vi "Measurement Logic Debug.vi"(8 "error in":errorcluster, 9 "measurement configuration":T4={"SERIAL CHANNEL"="SI1", "PATH TO CONFIGURATION SCRIPT"="\"C:\\dev\\scripts\\Image Receiver Scripts\\9296A_RAW8.cpp\"", "REF. CLOCK  (Hz)"=25000000.0, "POC SOURCE"=0, "CSI-2 DATA SOURCE"=0, "SI ACTIVE LANE CNT"=4, "PAYLOAD DATA TYPE"=enum."RAW 8", "INTERPRETATION"=1, "VIRTUAL CHANNEL"=0, "PATTERN"=0, "ALGORITHM"=0, "RIO HANDLER"="PXI1Slot2", "AUTO. VISION DEVICE"=0, "SERIAL (SI) CHANNEL"=1, "BITFILE"="PXIe_1487_4_In_4_Out_Acq_Tap.lvbitx", "SI CHANNELS"="SI0, S01"} {"SERIAL (SI) CHANNEL" items=["SI0", "SI1"]; "AUTO. VISION DEVICE" items=["PXI1Slot2", "PXI1Slot5"]; "ALGORITHM" items=["BILINEAR", "VNG"]; "PATTERN" items=["GB", "GR", "BG", "RG"]; "INTERPRETATION" items=["Grayscale", "Bayer", "RGB", "YUV422", "YUV420", "Legacy YUV420"]; "SI ACTIVE LANE CNT" items=["1 LANE"=1, "2 LANE"=2, "4 LANE"=4]; "CSI-2 DATA SOURCE" items=["CORRECTED", "RAW"]; "POC SOURCE" items=["NONE", "INTERNAL", "AUXILIARY"]}, 10 "measure call context in":refnum<class "Measure Call Context.lvclass">, 11 "user event out":refnum<user-event>) -> (0 "Error Out":errorcluster, 2 "measure call context out":refnum<class "Measure Call Context.lvclass">, 3 "measurement results":T1 {"BYTES ACQUIRED" format="%#.6p"})   [LabVIEW 2025]
doc: "Contains the core logic for executing the measurement."
uses:
  <vilib>/Plug-In SDKs/Measurements/Measure Call Context/Measure Call Context.lvclass
  <vilib>/rvi/interface/nirviCloseFPGA/nirviCloseFPGA.xnode
  Measurement Results.ctl
  Automotive Vision.lvclass
  deps/NI148X/Getting Started/Host/Acq/GettingStarted_Acq_148X_Host.lvlib
  deps/NI148X/Getting Started/Host/Common/GettingStarted_Common_148X_Host.lvlib
  <instrlib>/FlexRIO/API/Host/v1/NI FlexRIO API v1.lvlib
  <vilib>/vision/Image Controls.llb/IMAQ Image.ctl
  <instrlib>/FlexRIO/CSI-2/v2/Common/Types/LLP Data Type.ctl
  <instrlib>/FlexRIO/CSI-2/v2/Common/NI CSI-2 API Common v2.lvlib
  <instrlib>/FlexRIO/API/Host/v1/NI FlexRIO/API/Wait for PoC Safe to Disconnect Channels Array.vi
  <vilib>/FPGAPlugInAG/Dynamic/niLvFpga_Close_Dynamic.vi
  Measurement Configuration.ctl
panel:
  in  "Acquired Serial Input Channel Data":T2(tab)
  out "Source Rate (fps)(1st Display)":dbl
  out "Update Rate (fps)(1st Display)":dbl
  out "1st channel display":T3(plugin-control)
  out "Bytes Acquired (1st Channel)":i64 format="%#.6p"
  out "Packets Logged (1st Channel)":i64
  out "Source Rate (fps)(2nd Display)":dbl
  out "Update Rate (fps)(2nd Display)":dbl
  out "2nd channel display":T3(plugin-control)
  out "Packets Logged (2nd Channel)":i64
  out "Bytes Acquired (2nd Channel)":i64 format="%#.6p"
  out "Acquisition In Progress":bool
  out "Acquisition Duration (s)":dbl format="%.1f"
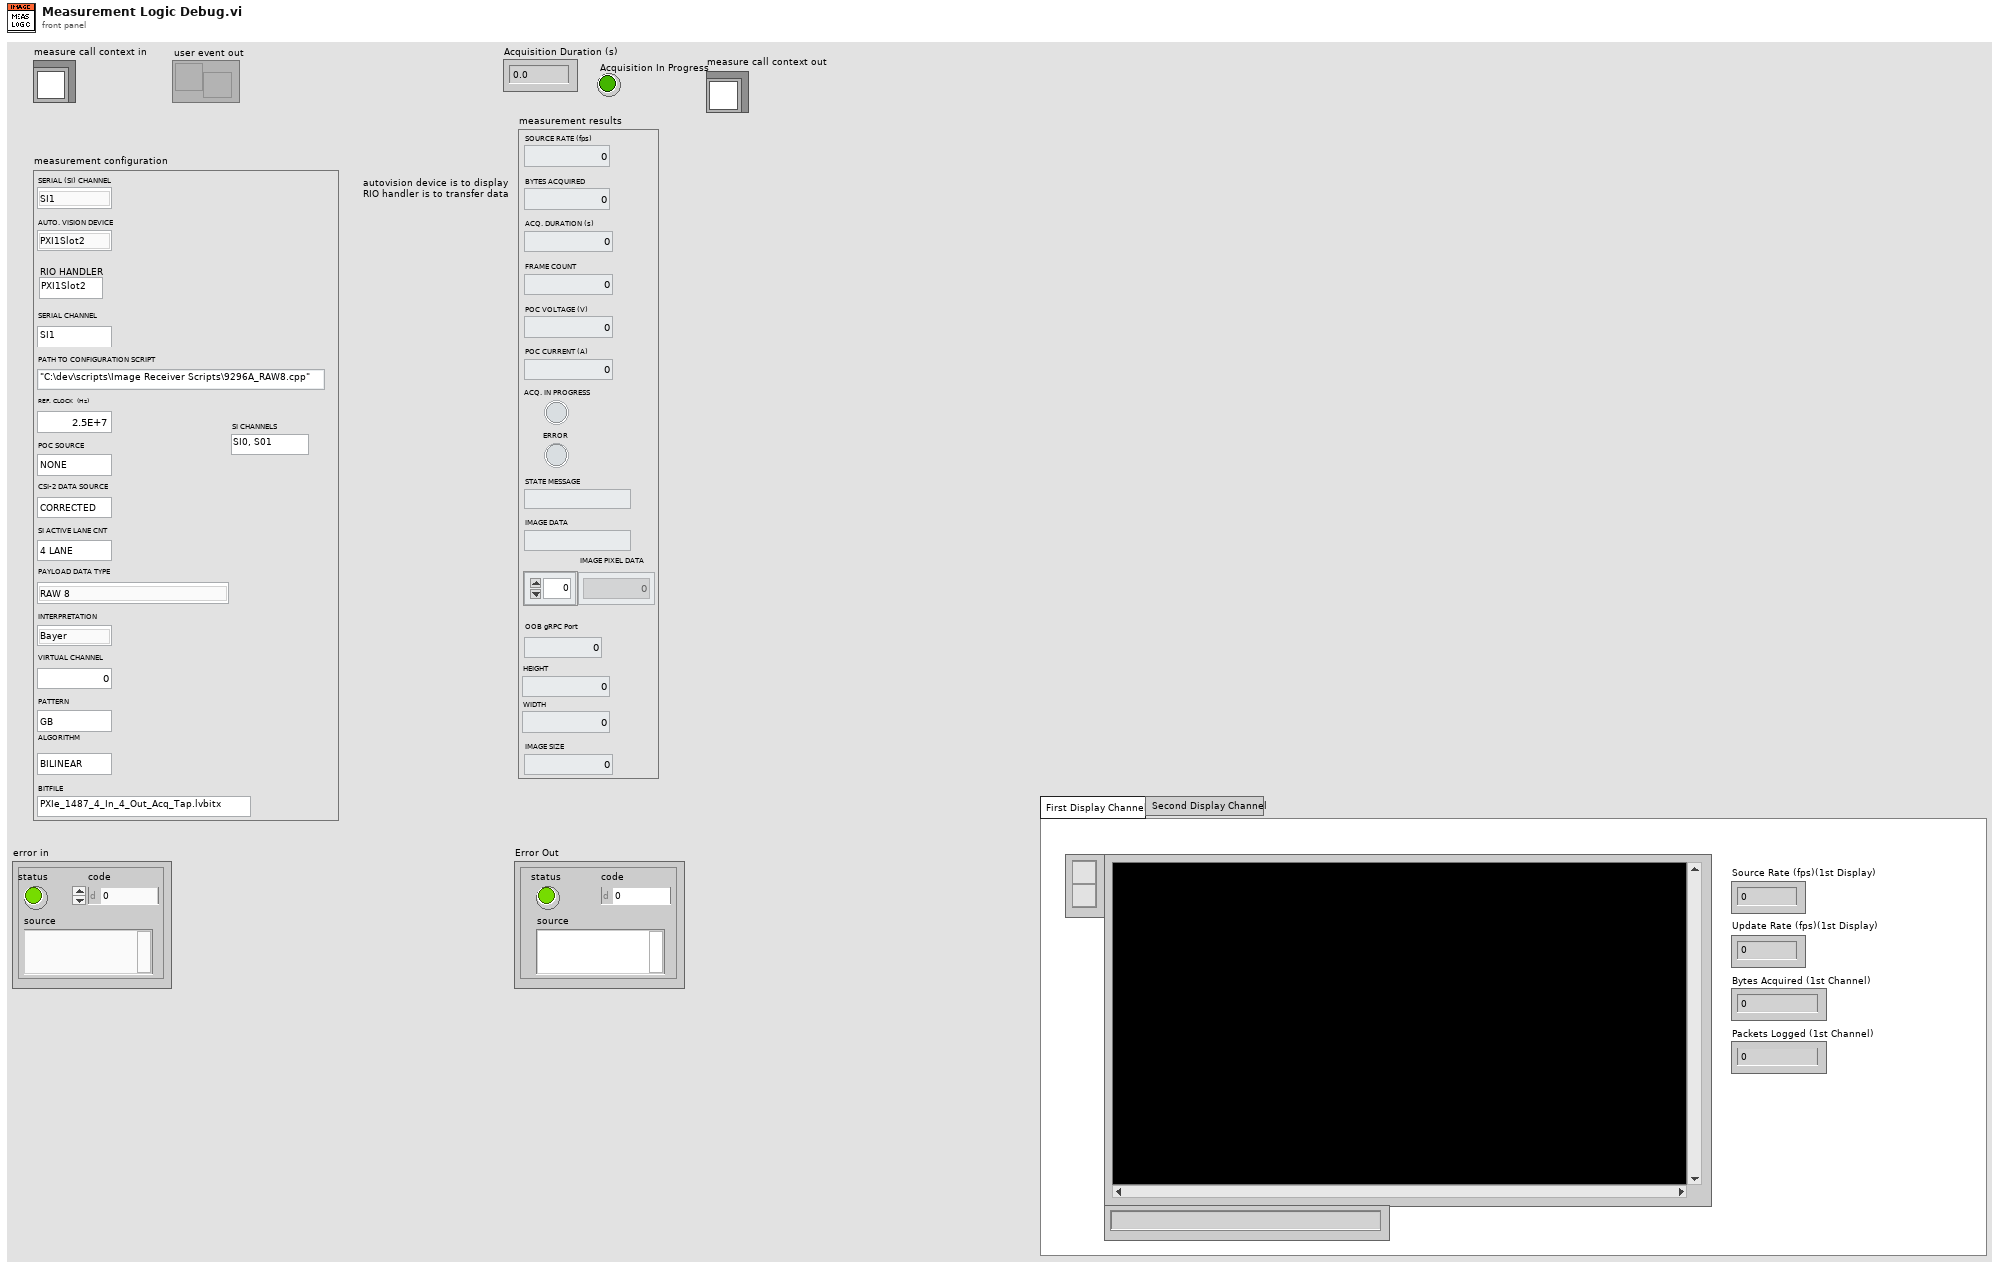
[diagram p1: front panel]
types:
  T1 = typedef "Automotive Vision.lvclass/Measurement Results.ctl" = cluster{"ACQ. IN PROGRESS":bool, "IMAGE PIXEL DATA":u32[], "ACQ. DURATION (s)":dbl, "SOURCE RATE (fps)":dbl, "BYTES ACQUIRED":u64, "FRAME COUNT":u64, "POC VOLTAGE (V)":dbl, "POC CURRENT (A)":dbl, "ERROR":bool, "STATE MESSAGE":string, "IMAGE DATA":string, "OOB gRPC Port":i32, "HEIGHT":u64, "WIDTH":u64, "IMAGE SIZE":u64}
  T2 = enum32{"First Display Channel", "Second Display Channel"}
  T3 = typedef "IMAQ Image.ctl" = refnum<image>
  T4 = typedef "Automotive Vision.lvclass/Measurement Configuration.ctl" = cluster{"SERIAL CHANNEL":string, "PATH TO CONFIGURATION SCRIPT":string, "REF. CLOCK  (Hz)":dbl, "POC SOURCE":u32, "CSI-2 DATA SOURCE":u32, "SI ACTIVE LANE CNT":u32, "PAYLOAD DATA TYPE":enum32{"Frame Start", "Frame End", "Line Start", "Line End", "End of Transmission", "Reserved 0", "Reserved 1", "Reserved 2", "Generic Short Packet 1", "Generic Short Packet 2", "Generic Short Packet 3", "Generic Short Packet 4", "Generic Short Packet 5", "Generic Short Packet 6", "Generic Short Packet 7", "Generic Short Packet 8", "Null", "Blanking Data", "Embedded 8-bit non Image Data", "Generic Long Packet 1", "Generic Long Packet 2", "Generic Long Packet 3", "Generic Long Packet 4", "Reserved 3", "YUV420 8-bit", "YUV420 10-bit", "Legacy YUV420 8-bit", "Reserved 4", "YUV420 8-bit Chroma Shifted", "YUV420 10-bit Chroma Shifted", "YUV422 8-bit", "YUV422 10-bit", "RGB444", "RGB555", "RGB565", "RGB666", "RGB888", "Reserved 5", "Reserved 6", "RAW 24", "RAW 6", "RAW 7", "RAW 8", "RAW 10", "RAW 12", "RAW 14", "RAW 16", "RAW 20", "User Defined 8-bit Data 1", "User Defined 8-bit Data 2", "User Defined 8-bit Data 3", "User Defined 8-bit Data 4", "User Defined 8-bit Data 5", "User Defined 8-bit Data 6", "User Defined 8-bit Data 7", "User Defined 8-bit Data 8", "USL Command", "Reserved 7", "Reserved 8", "Reserved 9", "Reserved 10", "Reserved 11", "Reserved 12", "LRTE EPD Spacer"}, "INTERPRETATION":u32, "VIRTUAL CHANNEL":u32, "PATTERN":u32, "ALGORITHM":u32, "RIO HANDLER":string, "AUTO. VISION DEVICE":u32, "SERIAL (SI) CHANNEL":u32, "BITFILE":string, "SI CHANNELS":string}
  T5 = typedef "NI CSI-2 API Common v2.lvlib/LLP Data Type.ctl" = enum8{"Frame Start", "Frame End", "Line Start", "Line End", "End of Transmission", "Reserved 0", "Reserved 1", "Reserved 2", "Generic Short Packet 1", "Generic Short Packet 2", "Generic Short Packet 3", "Generic Short Packet 4", "Generic Short Packet 5", "Generic Short Packet 6", "Generic Short Packet 7", "Generic Short Packet 8", "Null", "Blanking Data", "Embedded 8-bit non Image Data", "Generic Long Packet 1", "Generic Long Packet 2", "Generic Long Packet 3", "Generic Long Packet 4", "Reserved 3", "YUV420 8-bit", "YUV420 10-bit", "Legacy YUV420 8-bit", "Reserved 4", "YUV420 8-bit Chroma Shifted", "YUV420 10-bit Chroma Shifted", "YUV422 8-bit", "YUV422 10-bit", "RGB444", "RGB555", "RGB565", "RGB666", "RGB888", "Reserved 5", "Reserved 6", "RAW 24", "RAW 6", "RAW 7", "RAW 8", "RAW 10", "RAW 12", "RAW 14", "RAW 16", "RAW 20", "User Defined 8-bit Data 1", "User Defined 8-bit Data 2", "User Defined 8-bit Data 3", "User Defined 8-bit Data 4", "User Defined 8-bit Data 5", "User Defined 8-bit Data 6", "User Defined 8-bit Data 7", "User Defined 8-bit Data 8", "USL Command", "Reserved 7", "Reserved 8", "Reserved 9", "Reserved 10", "Reserved 11", "Reserved 12", "LRTE EPD Spacer"}
  T6 = typedef "GettingStarted_Common_148X_Host.lvlib/Serial Channel Configuration.ctl" = cluster{"Serial Channel":string, "FPGA Display Parameters":T7, "RAW Display Parameters":cluster{"Interpretation":T8, "Bayer Parameters":cluster{"Pattern":i32, "Algorithm":i32, "Red Gain":dbl, "Green Gain":dbl, "Blue Gain":dbl}}}
  T7 = typedef "NI CSI-2 API FPGA v2.lvlib/Display Parameters.ctl" = cluster{"virtual channel":fxp<+,4,4>, "payload data type":T5, "frame skip count":u16, "line skip count":u8, "pixel skip count":fxp<+,5,5>}
  T8 = typedef "GettingStarted_Common_148X_Host.lvlib/RAW Interpretation for Display.ctl" = enum16{"Grayscale", "Bayer", "RGB", "YUV422", "YUV420", "Legacy YUV420"}
  T9 = typedef "GettingStarted_Common_148X_Host.lvlib/Serial Channel Display Parameters.ctl" = cluster{"images":cluster{"grayscale":T3, "color":T3}, "RAW parameters":cluster{"interpretation":T8, "bayer parameters":cluster{"pattern":i32, "algorithm":i32, "red gain":dbl, "green gain":dbl, "blue gain":dbl}}}
  T10 = cluster{"Acquisition In Progress":refnum<vi>, "Acquisition Duration (s)":refnum<vi>, "Bytes Acquired (1st Channel)":refnum<vi>}
  T11 = typedef "Event Messenger-bool.lvlib/))Channel.ctl" = refnum<queue>
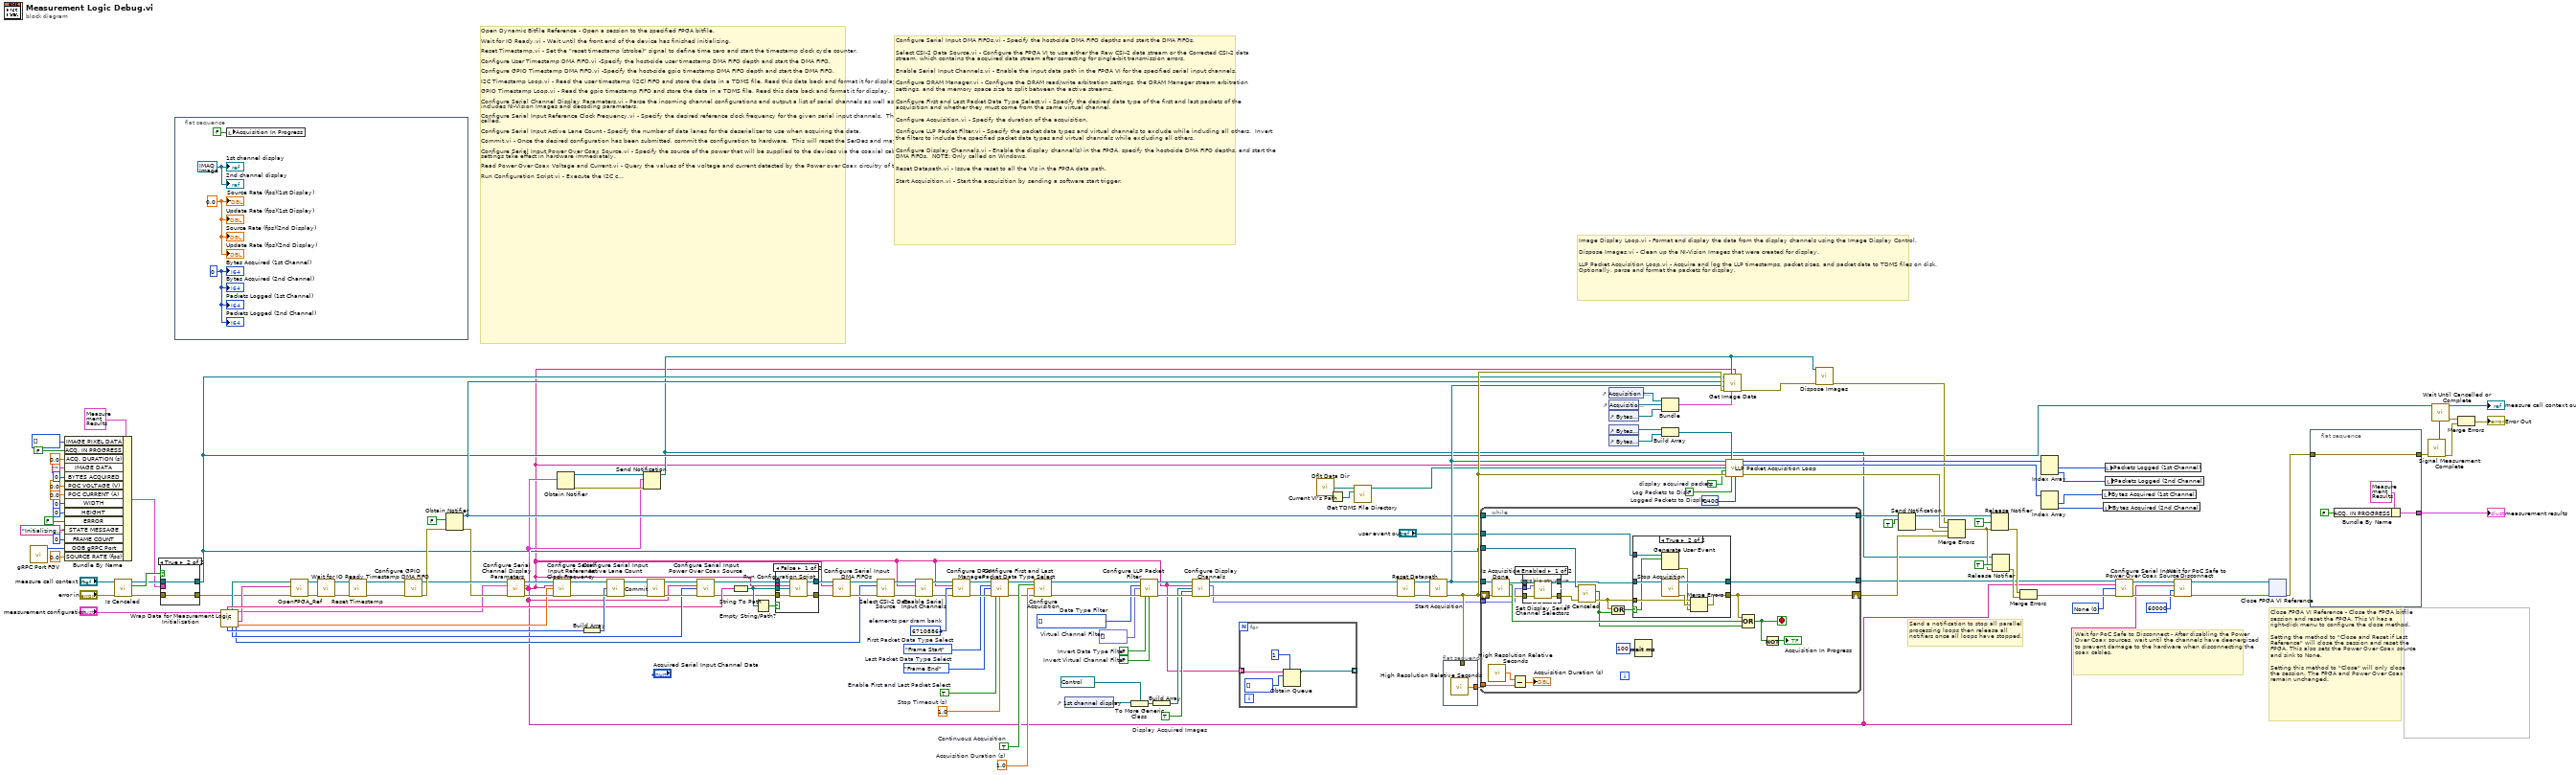
[diagram p0: block diagram]
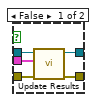
[diagram p2: hidden frame]
diagram:
  w78 = i64 1400  # Logged Packets to Display
  w102 = FALSE  # Log Packets to Disk
  w130 = FALSE  # Invert Virtual Channel Filter
  w131 = FALSE  # Invert Data Type Filter
  w132 = fxp<+,4,4>[] []  # Virtual Channel Filter
  w98 = TRUE  # Display Acquired Images
  w134 = T5[] [] items=["Frame Start", "Frame End", "Line Start", "Line End", "End of Transmission", "Reserved 0", "Reserved 1", "Reserved 2", "Generic Short Packet 1", "Generic Short Packet 2", "Generic Short Packet 3", "Generic Short Packet 4", "Generic Short Packet 5", "Generic Short Packet 6", "Generic Short Packet 7", "Generic Short Packet 8", "Null", "Blanking Data", "Embedded 8-bit non Image Data", "Generic Long Packet 1", "Generic Long Packet 2", "Generic Long Packet 3", "Generic Long Packet 4", "Reserved 3", "YUV420 8-bit", "YUV420 10-bit", "Legacy YUV420 8-bit", "Reserved 4", "YUV420 8-bit Chroma Shifted", "YUV420 10-bit Chroma Shifted", "YUV422 8-bit", "YUV422 10-bit", "RGB444", "RGB555", "RGB565", "RGB666", "RGB888", "Reserved 5", "Reserved 6", "RAW 24", "RAW 6", "RAW 7", "RAW 8", "RAW 10", "RAW 12", "RAW 14", "RAW 16", "RAW 20", "User Defined 8-bit Data 1", "User Defined 8-bit Data 2", "User Defined 8-bit Data 3", "User Defined 8-bit Data 4", "User Defined 8-bit Data 5", "User Defined 8-bit Data 6", "User Defined 8-bit Data 7", "User Defined 8-bit Data 8", "USL Command", "Reserved 7", "Reserved 8", "Reserved 9", "Reserved 10", "Reserved 11", "Reserved 12", "LRTE EPD Spacer"]  # Data Type Filter
  w137 = 1.0  # Acquisition Duration (s)
  w140 = TRUE  # Continuous Acquisition
  w120 = 1.0  # Stop Timeout (s)
  w121 = TRUE  # Enable First and Last Packet Select
  w118 = LLP_Data_Type."Frame End"  # Last Packet Data Type Select
  w119 = LLP_Data_Type."Frame Start"  # First Packet Data Type Select
  w59 = 0 items=["None", "Internal", "Auxiliary"] ("power over coax source")
  w79 = TRUE  # display acquired packets
  w146 = u32 67108864  # elements per dram bank
  # "Wait for PoC Safe to Disconnect - After disabling the Power Over Coax sources, wait until the channels have deenergized to prevent damage to the hardware when disconnecting the coax cables."
  # "Send a notification to stop all parallel processing loops then release all notifiers once all loops have stopped."
  # "Image Display Loop.vi - Format and display the data from the display channels using the Image Display Control.   \n\nDispose Images.vi - Clean up the NI-Vision Images that were created for display.\n\nLLP Packet Acquisition Loop.vi - Acquire and log the LLP timestamps, packet sizes, and packet data to TDMS files on disk.  Optionally, parse and format the packets for display."
  # "Configure Serial Input DMA FIFOs.vi - Specify the host-side DMA FIFO depths and start the DMA FIFOs.\n\nSelect CSI-2 Data Source.vi - Configure the FPGA VI to use either the Raw CSI-2 data stream or the Corrected CSI-2 data stream, which contains the acquired data stream after correcting for single-bit transmission errors.\n\nEnable Serial Input Channels.vi - Enable the input data path in the FPGA VI for the specified serial input channels.\n\nConfigure DRAM Manager.vi - Configure the DRAM read/write arbitration settings, the DRAM Manager stream arbitration settings, and the memory space size to split between the active streams.\n\nConfigure First and Last Packet Data Type Select.vi - Specify the desired data type of the first and last packets of the acquisition and whether they must come from the same virtual channel.\n\nConfigure Acquisition.vi - Specify the duration of the acquisition.\n\nConfigure LLP Packet Filter.vi - Specify the packet data types and virtual channels to exclude while including all others.  Invert the filters to include the specified packet data types and virtual channels while excluding all others.\n\nConfigure Display Channels.vi - Enable the display channel(s) in the FPGA, specify the host-side DMA FIFO depths, and start the DMA FIFOs.  NOTE: Only called on Windows. \n\nReset Datapath.vi - Issue the reset to all the VIs in the FPGA data path.\n\nStart Acquisition.vi - Start the acquisition by sending a software start trigger."
  # "Close FPGA VI Reference - Close the FPGA bitfile session and reset the FPGA. This VI has a right-click menu to configure the close method. \n\nSetting the method to \"Close and Reset if Last Reference\" will close the session and reset the FPGA. This also sets the Power Over Coax source and sink to None.\n\nSetting this method to \"Close\" will only close the session. The FPGA and Power Over Coax remain unchanged."
  # "Open Dynamic Bitfile Reference - Open a session to the specified FPGA bitfile.\n\nWait for IO Ready.vi - Wait until the front end of the device has finished initializing.\n\nReset Timestamp.vi - Set the \"reset timestamp (strobe)\" signal to define time zero and start the timestamp clock cycle counter.\n\nConfigure User Timestamp DMA FIFO.vi -Specify the host-side user timestamp DMA FIFO depth and start the DMA FIFO.\n\nConfigure GPIO Timestamp DMA FIFO.vi -Specify the host-side gpio timestamp DMA FIFO depth and start the DMA FIFO.\n\nI2C Timestamp Loop.vi - Read the user timestamp (I2C) FIFO and store the data in a TDMS file. Read this data back and format it for display.\n\nGPIO Timestamp Loop.vi - Read the gpio timestamp FIFO and store the data in a TDMS file. Read this data back and format it for display.\n\nConfigure Serial Channel Display Parameters.vi - Parse the incoming channel configurations and output a list of serial channels as well as a list of serial channel display parameters, which includes NI-Vision Images and decoding parameters.\n\nConfigure Serial Input Reference Clock Frequency.vi - Specify the desired reference clock frequency for the given serial input channels.  These settings do not take effect until Commit.vi is called.\n\nConfigure Serial Input Active Lane Count - Specify the number of data lanes for the deserializer to use when acquiring the data. \n\nCommit.vi - Once the desired configuration has been submitted, commit the configuration to hardware.  This will reset the SerDes and may cause GPIO lines to toggle. \n\nConfigure Serial Input Power Over Coax Source.vi - Specify the source of the power that will be supplied to the devices via the coaxial cables attached to the given serial input channels.  These settings take effect in hardware immediately.\n\nRead Power Over Coax Voltage and Current.vi - Query the values of the voltage and current detected by the Power over Coax circuitry of the given serial channels.\n\nRun Configuration Script.vi - Execute the I2C commands in the specified script file for the given serial channels.  The script is used to configure the serializer, deserializer, or other I2C slave device, such as the image sensor."
  n1 = call "gRPC Port FGV.vi"() -> ("Listening Port out"=w31:i32)  [unwired: 11 in]
  n2 = Bundle By Name(cluster=T1 {"ACQ. IN PROGRESS"=FALSE, "IMAGE PIXEL DATA"=[], "ACQ. DURATION (s)"=0.0, "SOURCE RATE (fps)"=0.0, "BYTES ACQUIRED"=0, "FRAME COUNT"=0, "POC VOLTAGE (V)"=0.0, "POC CURRENT (A)"=0.0, "ERROR"=FALSE, "STATE MESSAGE"="", "IMAGE DATA"="", "OOB gRPC Port"=0, "HEIGHT"=0, "WIDTH"=0, "IMAGE SIZE"=0} ("Measurement Results"), "IMAGE PIXEL DATA"=u32[] [], "ACQ. IN PROGRESS"=FALSE, "ACQ. DURATION (s)"=0.0, "IMAGE DATA"="", "BYTES ACQUIRED"=u64 0, "POC VOLTAGE (V)"=0.0, "POC CURRENT (A)"=0.0, "WIDTH"=u64 0, "HEIGHT"=u64 0, "ERROR"=FALSE, "STATE MESSAGE"="Initializing...", "FRAME COUNT"=u64 0, "OOB gRPC Port"=w31, "SOURCE RATE (fps)"=0.0) -> (w27:T1)
  n3 = call <vilib>:"Is Canceled.vi"("error in"="error in", "measure call context in"="measure call context in") -> ("error out"=w30:errorcluster, "is canceled?"=w29:bool, "measure call context out"=w28:refnum<class "Measure Call Context.lvclass">)  [unwired: 7 in]
  n4 = case shown="True" w29 {
    tunnel: w27 -> [w155 _]
    tunnel: [w154 w157] -> w24
    tunnel: w28 -> [w153 w156]
    tunnel: w30 -> [w152 w157]
    tunnel: [w151 w156] -> w9
    frame False {
      n5 = call <vilib>:"Update Results.vi"("error in"=w152, "measurement results"=w155, "measure call context in"=w153) -> ("error out"=w154:errorcluster, "measure call context out"=w151:refnum<class "Measure Call Context.lvclass">)  [unwired: 7 in]
    }
    frame True {
    }
  }
  n6 = flat-sequence {
    frame #0 {
      w159 = i64 0 ("Number of Packets Acquired (1st Channel)")
      w160 = 0.0 ("display fps (2nd display)")
      w161 = T3 refnum ("first channel display")
      n7 = local write "Acquisition In Progress"(FALSE ("Acquisition In Progress")) -> ()
      "1st channel display" <- w161
      "2nd channel display" <- w161
      "Update Rate (fps)(1st Display)" <- w160
      "Update Rate (fps)(2nd Display)" <- w160
      "Packets Logged (1st Channel)" <- w159
      "Packets Logged (2nd Channel)" <- w159
      "Source Rate (fps)(1st Display)" <- w160
      "Source Rate (fps)(2nd Display)" <- w160
      "Bytes Acquired (1st Channel)" <- w159
      "Bytes Acquired (2nd Channel)" <- w159
    }
  }
  n8 = call "Wrap Data for Measurement Logic Initialization.vi"("measurement configuration"="measurement configuration") -> ("REF. CLOCK  (Hz)"=w49:dbl, "RIO HANDLER"=w45:string, "CSI-2 DATA SOURCE"=w50:u32, "Serial Input Configuration"=w38:T6[], "POC SOURCE"=w51:u32, "appended path"=w44:path, "SI ACTIVE LANE CNT"=w52:u32, "PATH TO CONFIGURATION SCRIPT"=w48:string)  [unwired: 3 in]
  n9 = call "OpenFPGA_Ref.vi"("error in"=w24, "RIO HANDLER"=w45, "Bitfile path"=w44) -> ("error out"=w39:errorcluster, "Refnum out"=w133:refnum<k20>)  [unwired: 7 in]
  n10 = call <instrlib>:"Wait for IO Ready.vi"("fpga interface in"=w133, "error in"=w39) -> ("fpga interface out"=w95:refnum<k20>, "error out"=w96:errorcluster)  [unwired: 10 in, 2 out]
  n11 = call "Reset Timestamp.vi"("fpga interface in"=w95, "error in (no error)"=w96) -> ("fpga interface out"=w5:refnum<k20>, "error out"=w4:errorcluster)  [unwired: 12 in]
  n12 = call "Configure GPIO Timestamp DMA FIFO.vi"("fpga interface in"=w5, "error in (no error)"=w4) -> ("fpga interface out"=w83:refnum<k20>, "error out"=w85:errorcluster)  [unwired: 12 in]
  n13 = Obtain Notifier(notification data type=FALSE ("result"), error in (no error)=w85) -> (notifier out=w71:refnum<notifier>, error out=w82:errorcluster)  [unwired: 2 in, 1 out]
  n14 = call "Configure Serial Channel Display Parameters.vi"("fpga interface in"=w83, "serial channel configurations"=w38, "error in (no error)"=w82) -> ("fpga interface out"=w110:refnum<k20>, "serial channel display parameters"=w68:T9[], "serial channels"=w2:string[], "error out"=w109:errorcluster)  [unwired: 9 in]
  n15 = call "Configure Serial Input Reference Clock Frequency.vi"("fpga interface in"=w110, "serial input channels"=w2, "serial input reference clock frequency (Hz)"=w49, "error in (no error)"=w109) -> ("fpga interface out"=w76:refnum<k20>, "error out"=w75:errorcluster)  [unwired: 10 in]
  n16 = Obtain Notifier(notification data type=w68) -> (notifier out=w70:refnum<notifier>, error out=w69:errorcluster)  [unwired: 3 in, 1 out]
  n17 = Build Array(w52) -> (w72:u32[])
  n18 = call "Configure Serial Input Active Lane Count.vi"("fpga interface in"=w76, "serial input active lane counts"=w72, "error in (no error)"=w75) -> ("fpga interface out"=w74:refnum<k20>, "error out"=w73:errorcluster)  [unwired: 11 in]
  n19 = Send Notification(notification=w68, notifier=w70, error in (no error)=w69) -> (notifier out=w8:refnum<notifier>)  [unwired: 1 out]
  n20 = call <instrlib>:"Commit.vi"("fpga interface in"=w74, "error in"=w73) -> ("fpga interface out"=w135:refnum<k20>, "error out"=w136:errorcluster)  [unwired: 12 in]
  n21 = call "Configure Serial Input Power Over Coax Source.vi"("fpga interface in"=w135, "serial input channels"=w2, "power over coax source"=w51, "error in (no error)"=w136) -> ("fpga interface out"=w33:refnum<k20>, "error out"=w32:errorcluster)  [unwired: 9 in, 1 out]
  n22 = String To Path(string=w48) -> (path=w47:path)
  n23 = Empty String/Path?(string/path=w47) -> (empty?=w97:bool)
  n24 = case shown="False" w97 {
    tunnel: [w167 w168] -> w144
    tunnel: [w166 w169] -> w139
    tunnel: w32 -> [w165 w168]
    tunnel: w33 -> [w164 w169]
    tunnel: w2 -> [w163 _]
    tunnel: w47 -> [w162 _]
    frame False {
      n25 = call "Run Configuration Script.vi"("fpga interface in"=w164, "serial channels"=w163, "configuration script"=w162, "error in (no error)"=w165) -> ("fpga interface out"=w166:refnum<k20>, "error out"=w167:errorcluster)  [unwired: 10 in]
    }
    frame True {
    }
  }
  n26 = call "Configure Serial Input DMA FIFOs.vi"("fpga interface in"=w139, "serial channels"=w2, "error in (no error)"=w144) -> ("fpga interface out"=w129:refnum<k20>, "error out"=w126:errorcluster)  [unwired: 11 in]
  n27 = call "Select CSI-2 Data Source.vi"("fpga interface in"=w129, "csi-2 data source"=w50, "error in (no error)"=w126) -> ("fpga interface out"=w128:refnum<k20>, "error out"=w127:errorcluster)  [unwired: 11 in]
  n28 = call "Enable Serial Input Channels.vi"("fpga interface in"=w128, "serial input channels"=w2, "error in (no error)"=w127) -> ("fpga interface out"=w138:refnum<k20>, "error out"=w145:errorcluster)  [unwired: 11 in]
  n29 = call "Configure DRAM Manager.vi"("fpga interface in"=w138, "serial channels"=w2, "elements per dram bank"=w146, "error in (no error)"=w145) -> ("fpga interface out"=w122:refnum<k20>, "error out"=w125:errorcluster)  [unwired: 10 in]
  n30 = call "Configure First and Last Packet Data Type Select.vi"("fpga interface in"=w122, "first packet data type select"=w119, "last packet data type select"=w118, "error in (no error)"=w125, "enable first and last packet select"=w121, "stop timeout (s)"=w120) -> ("fpga interface out"=w123:refnum<k20>, "error out"=w124:errorcluster)  [unwired: 8 in]
  n31 = call "Configure Acquisition.vi"("fpga interface in"=w123, "continuous acquisition (T)"=w140, "acquisition duration (s)"=w137, "error in (no error)"=w124) -> ("fpga interface out"=w141:refnum<k20>, "error out"=w142:errorcluster)  [unwired: 10 in]
  n32 = control-ref of="1st channel display"() -> (w35:refnum<vi>)
  n33 = To More Generic Class(target class=refnum<vi> refnum ("image display reference"), reference=w35) -> (generic class reference=w37:refnum<vi>)
  n34 = call "Configure LLP Packet Filter.vi"("fpga interface in"=w141, "data type filter"=w134, "virtual channel filter"=w132, "error in (no error)"=w142, "invert data type filter"=w131, "invert virtual channel filter"=w130) -> ("fpga interface out"=w111:refnum<k20>, "error out"=w108:errorcluster)  [unwired: 8 in]
  n35 = Build Array(w37) -> (w34:refnum<vi>[])
  n36 = call "Configure Display Channels.vi"("fpga interface in"=w111, "serial channels"=w2, "display references in"=w34, "enable image display"=w98, "error in (no error)"=w108) -> ("fpga interface out"=w107:refnum<k20>, "display serial channels"=w3:fxp<+,3,3>[], "error out"=w106:errorcluster)  [unwired: 7 in, 1 out]
  n37 = for {
    tunnel: w2 -> [w173] mode=indexing
    tunnel: [w171] -> _ mode=indexing
    n38 = Obtain Queue(max queue size (-1, unlimited)=1, name (unnamed)=w173, element data type=u32[] [] ("Image Pixels (U32)")) -> (queue out=w171:refnum<queue>)  [unwired: 2 in, 2 out]
  }
  n39 = call <vilib>:"Dflt Data Dir.vi"() -> ("App:Default Data Directory"=w46:path)
  n40 = Current VI's Path() -> (path=w114:path)
  n41 = call "Get TDMS File Directory.vi"("tdms file directory in"=w46, "calling vi path"=w114) -> ("tdms file directory out"=w81:path)  [unwired: 13 in]
  n42 = call "Reset Datapath.vi"("fpga interface in"=w107, "error in (no error)"=w106) -> ("fpga interface out"=w143:refnum<k20>, "error out"=w84:errorcluster)  [unwired: 12 in]
  n43 = call "Start Acquisition.vi"("fpga interface in"=w143, "error in (no error)"=w84) -> ("fpga interface out"=w93:refnum<k20>, "error out"=w94:errorcluster)  [unwired: 12 in]
  n44 = flat-sequence {
    tunnel: [w174] -> w115
    tunnel: w94 -> [_]
    frame #0 {
      n45 = call <vilib>:"High Resolution Relative Seconds.vi"() -> ("relative seconds"=w174:dbl)
    }
  }
  n46 = while {
    shift-right: [w183] -> w77
    shift-left: w94 -> [w190]
    tunnel: w93 -> [w192]
    tunnel: w115 -> [w193]
    tunnel: w71 -> [w189]
    tunnel: [w189] -> w90
    tunnel: [w184] -> w63
    tunnel: w9 -> [w188]
    tunnel: "user event out" -> [w180]
    tunnel: w3 -> [w175]
    stop <- w191 stop-if-true
    n47 = call <vilib>:"High Resolution Relative Seconds.vi"() -> ("relative seconds"=w194:dbl)
    n48 = call "Is Acquisition Done.vi"("fpga interface in"=w192, "error in (no error)"=w190) -> ("fpga interface out"=w179:refnum<k20>, "acquisition done"=w196:bool, "error out"=w177:errorcluster)  [unwired: 11 in]
    n49 = Subtract(x=w194, y=w193) -> (x-y=→"Acquisition Duration (s)":dbl)
    n50 = disable-structure shown="Enabled" {
      disable-tunnel: w179 -> [w201 w203]
      disable-tunnel: [w200 w203] -> w178
      disable-tunnel: w177 -> [w199 w202]
      disable-tunnel: [w198 w202] -> w176
      disable-tunnel: w175 -> [w197 _]
      frame Enabled {
        n51 = call "Set Display Serial Channel Selectors.vi"("fpga interface in"=w201, "display serial channel selectors"=w197, "error in (no error)"=w199) -> ("fpga interface out"=w200:refnum<k20>, "error out"=w198:errorcluster)  [unwired: 11 in]
      }
      frame Disabled {
      }
    }
    n52 = call <vilib>:"Is Canceled.vi"("error in"=w176, "measure call context in"=w188) -> ("error out"=w186:errorcluster, "is canceled?"=w182:bool)  [unwired: 7 in, 1 out]
    n53 = Compound Arithmetic op=OR(w186, w182) -> (w181:bool)
    n54 = case shown="True" w181 {
      selector: w181 -> [_ w207]
      tunnel: [w205 w210] -> w183
      tunnel: w186 -> [w205 w209]
      tunnel: [w204 w212] -> w184
      tunnel: w178 -> [w204 w211]
      tunnel: w180 -> [_ w208]
      frame False {
      }
      frame True {
        n55 = Generate User Event(user event=w208, event data cluster=w207) -> (error out=w206:errorcluster)  [unwired: 2 in, 1 out]
        n56 = call "Stop Acquisition.vi"("fpga interface in"=w211) -> ("fpga interface out"=w212:refnum<k20>, "error out"=w213:errorcluster)  [unwired: 13 in]
        n57 = Merge Errors(w209, w213, w206) -> (w210:errorcluster)
      }
    }
    n58 = Wait (ms)(milliseconds to wait=u32 100) -> ()  [unwired: 1 out]
    n59 = Compound Arithmetic op=OR(w183, w196, w182) -> (w191:bool)
    n60 = Not(x=w191) -> (.not. x?=→"Acquisition In Progress":bool)
  }
  n61 = control-ref of="Acquisition In Progress"() -> (w43:refnum<vi>)
  n62 = control-ref of="Acquisition Duration (s)"() -> (w42:refnum<vi>)
  n63 = control-ref of="Bytes Acquired (1st Channel)"() -> (w41:refnum<vi>)
  n64 = control-ref of="Bytes Acquired (1st Channel)"() -> (w117:refnum<vi>)
  n65 = control-ref of="Bytes Acquired (2nd Channel)"() -> (w116:refnum<vi>)
  n66 = Bundle("Acquisition In Progress"=w43, "Acquisition Duration (s)"=w42, "Bytes Acquired (1st Channel)"=w41) -> (w40:T10)  [unwired: 1 in]
  n67 = Build Array(w117, w116) -> (w113:refnum<vi>[])
  n68 = call "Get Image Data.vi"("serial channels"=w2, "References"=w40, "serial channel display parameters"=w8, "error in (no error)"=w94, "fpga interface in"=w93, "Acquisition Stopped Notifier"=w71, "Measure Call Context in"=w9) -> ("error out"=w103:errorcluster)  [unwired: 4 in]
  n69 = call "LLP Packet Acquisition Loop.vi"("fpga interface in"=w93, "bytes acquired references"=w113, "Serial Channels"=w2, "tdms file directory"=w81, "display acquired packets"=w79, "error in"=w94, "log to disk"=w102, "num packets to read"=w78) -> ("number of packets acquired"=w112:i64[], "number of bytes acquired"=w101:i64[], "error out"=w91:errorcluster)  [unwired: 4 in, 1 out]
  n70 = call "Dispose Images.vi"("raw display notifier"=w8, "error in (no error)"=w103) -> ("error out"=w80:errorcluster)  [unwired: 13 in]
  n71 = Send Notification(notification=TRUE, notifier=w90) -> (notifier out=w89:refnum<notifier>, error out=w88:errorcluster)  [unwired: 1 in]
  n72 = Merge Errors(w80, w91, w88, w77) -> (w66:errorcluster)
  n73 = Release Notifier(notifier=w89, force destroy? (F)=TRUE, error in (no error)=w66) -> (error out=w65:errorcluster)  [unwired: 2 out]
  n74 = Release Notifier(notifier=w8, force destroy? (F)=TRUE, error in (no error)=w66) -> (error out=w64:errorcluster)  [unwired: 2 out]
  n75 = Merge Errors(w65, w64) -> (w62:errorcluster)
  n76 = Index Array(array=w112) -> (element #1=w105:i64, element #2=w104:i64)  [unwired: 2 in]
  n77 = Index Array(array=w101) -> (element #1=w100:i64, element #2=w99:i64)  [unwired: 2 in]
  n78 = local write "Bytes Acquired (1st Channel)"(w100) -> ()
  n79 = local write "Bytes Acquired (2nd Channel)"(w99) -> ()
  n80 = local write "Packets Logged (1st Channel)"(w105) -> ()
  n81 = local write "Packets Logged (2nd Channel)"(w104) -> ()
  n82 = call "Configure Serial Input Power Over Coax Source.vi"("fpga interface in"=w63, "serial input channels"=w2, "power over coax source"=w59, "error in (no error)"=w62) -> ("fpga interface out"=w57:refnum<k20>, "error out"=w58:errorcluster)  [unwired: 9 in, 1 out]
  n83 = call-poly <instrlib>:"Wait for PoC Safe to Disconnect.vi"("error in"=w58, "Timeout (ms)"=60000 ("Wait for Safe to Disconnect Timeout (ms)"), "Channels"=w2, "fpga interface in"=w57) -> ("error out"=w61:errorcluster, "fpga interface out"=w60:refnum<k20>)  [unwired: 6 in]
  n84 = xnode ("Close FPGA VI Reference")("FPGA VI Reference In"=w60, "error in"=w61) -> ("error out"=w53:errorcluster)
  n85 = flat-sequence {
    tunnel: [w216] -> w54
    tunnel: w53 -> [w214]
    tunnel: [w214] -> w7
    frame #0 {
      n86 = Bundle By Name(cluster=T1 {"ACQ. IN PROGRESS"=FALSE, "IMAGE PIXEL DATA"=[], "ACQ. DURATION (s)"=0.0, "SOURCE RATE (fps)"=0.0, "BYTES ACQUIRED"=0, "FRAME COUNT"=0, "POC VOLTAGE (V)"=0.0, "POC CURRENT (A)"=0.0, "ERROR"=FALSE, "STATE MESSAGE"="", "IMAGE DATA"="", "OOB gRPC Port"=0, "HEIGHT"=0, "WIDTH"=0, "IMAGE SIZE"=0} ("Measurement Results"), "ACQ. IN PROGRESS"=FALSE) -> (w216:T1)
    }
  }
  n87 = call "Signal Measurement Complete.vi"("error in (no error)"=w7) -> ("error out"=w148:errorcluster, "done channel"=w149:T11)  [unwired: 9 in]
  n88 = call "Wait Until Cancelled or Complete.vi"("done channel"=w149, "measure call context in"=w9) -> ("error out"=w147:errorcluster, "measure call context out"=→"measure call context out":refnum<class "Measure Call Context.lvclass">)  [unwired: 8 in]
  n89 = Merge Errors(w147, w148) -> (→"Error Out":errorcluster)
  "measurement results" <- w54
